vi "Create_AO_Signal.vi"(8 "error in":errorcluster, 10 "AO Amplitude":dbl(slide) min=0.0 max=100.0 step=1.0 scale=0.0..100.0, 11 "ON / OFF":bool=TRUE) -> (0 "error out":errorcluster, 3 "WF":dbl[](array[numeric]))   [LabVIEW 2025]
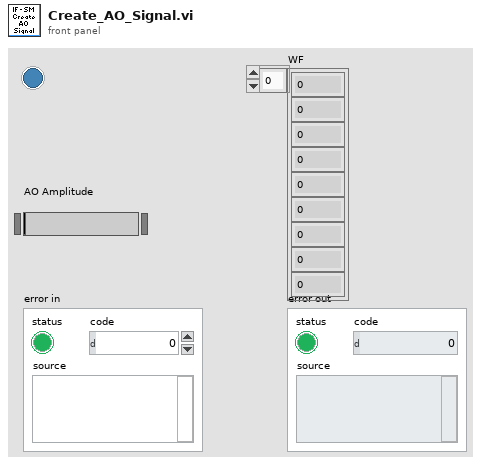
[diagram p1: front panel]
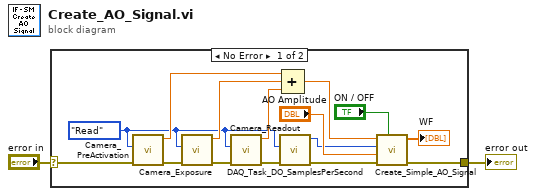
[diagram p0: block diagram]
diagram:
  n1 = case shown="No Error" "error in" {
    selector: "error in" -> [w17 w18]
    tunnel: [w6 w18] -> w1
    frame No Error {
      w3 = enum16{"Init", "Write", "Read"}."Read" ("Action")
      n2 = call "Camera_PreActivation.vi"("error in"=w17, "Action"=w3) -> ("error out"=w16:errorcluster, "Camera_PreActivation"=w11:dbl)  [unwired: 8 in]
      n3 = call "Camera_Exposure.vi"("error in"=w16, "Action"=w3) -> ("error out"=w15:errorcluster, "Exposure (s)"=w10:dbl)  [unwired: 8 in]
      n4 = call "Camera_Readout.vi"("error in"=w15, "Action"=w3) -> ("error out"=w14:errorcluster, "Camera_Readout"=w4:dbl)  [unwired: 8 in]
      n5 = call "DAQ_Task_DO_SamplesPerSecond.vi"("error in"=w14, "Action"=w3) -> ("error out"=w13:errorcluster, "DO_Task_SamplesPerSec"=w7:u32)  [unwired: 8 in]
      n6 = Compound Arithmetic op=ADD(w11, w10, w4) -> (w9:dbl)
      n7 = call "Create_Simple_AO_Signal.vi"("On/OFF"="ON / OFF", "error in"=w13, "Amplitude"="AO Amplitude", "Samples / s (10000)"=w7, "Time (s)"=w9) -> ("error out"=w6:errorcluster, "Signal"=→"WF":dbl[])  [unwired: 5 in]
    }
    frame Error {
    }
  }
  "error out" <- w1
